vi "PROIECT4.vi"() -> ()   [LabVIEW 2021]
uses:
  <vilib>/express/express analysis/Spectral/Block/exnSpectralBlock spectral measurements RMS poly.vi
  <vilib>/express/express analysis/Spectral/Block/exnSpectralBlock spectral measurements RMS WFM.vi
  <vilib>/express/express analysis/Spectral/XNode/ExpressSpectralMeasurementsBlockNode.xnode
  <vilib>/measure/NI_MABase.lvlib
panel:
  in  "AMPLITUDINE":dbl(slide) scale=0.0..10.0
  in  "?":T1(radio)
  out "?":dbl
  out "?":dbl
  out "?":dbl
  out "GRAFIC SEMNAL":waveform(dbl)(graph)
  out "ANALIZA SPECTRALA":cluster{"f0":dbl, "df":dbl, "magnitude":dbl[]}(graph)
  in  "?":bool
  in  "FAZA":dbl(slide) scale=0.0..360.0
  in  "FRECVENTA":dbl(knob) scale=0.0..100.0
  # "amplitudine"
  # "faza"
  # "frecventa"
  # "ON/OFF"
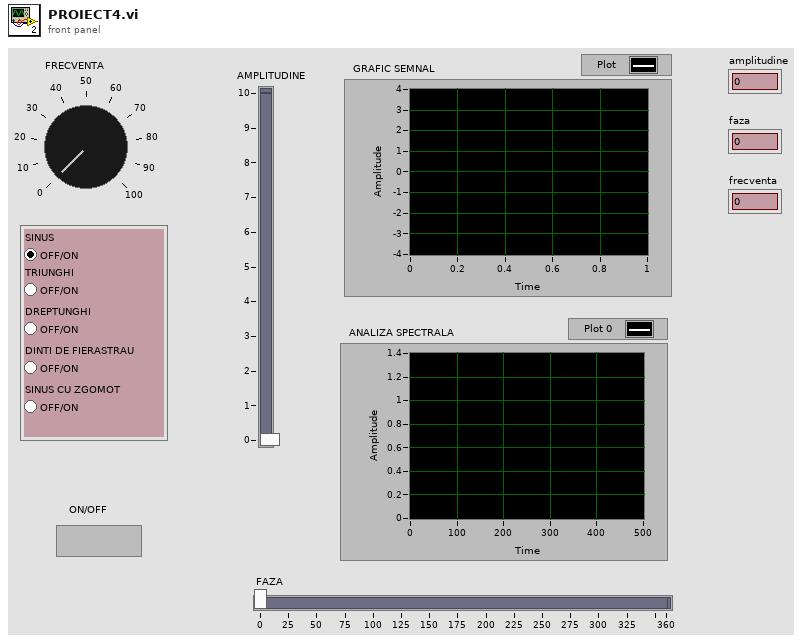
[diagram p1: front panel]
types:
  T1 = enum32{"SINUS", "TRIUNGHI", "DREPTUNGHI", "DINTI DE FIERASTRAU", "SINUS CU ZGOMOT"}
  T2 = cluster{"averaging mode":u16, "weighting mode":u16, "number of averages":u32}
  T3 = cluster{"dB On (F)":bool, "unwrap phase (F)":bool, "convert to degree (F)":bool}
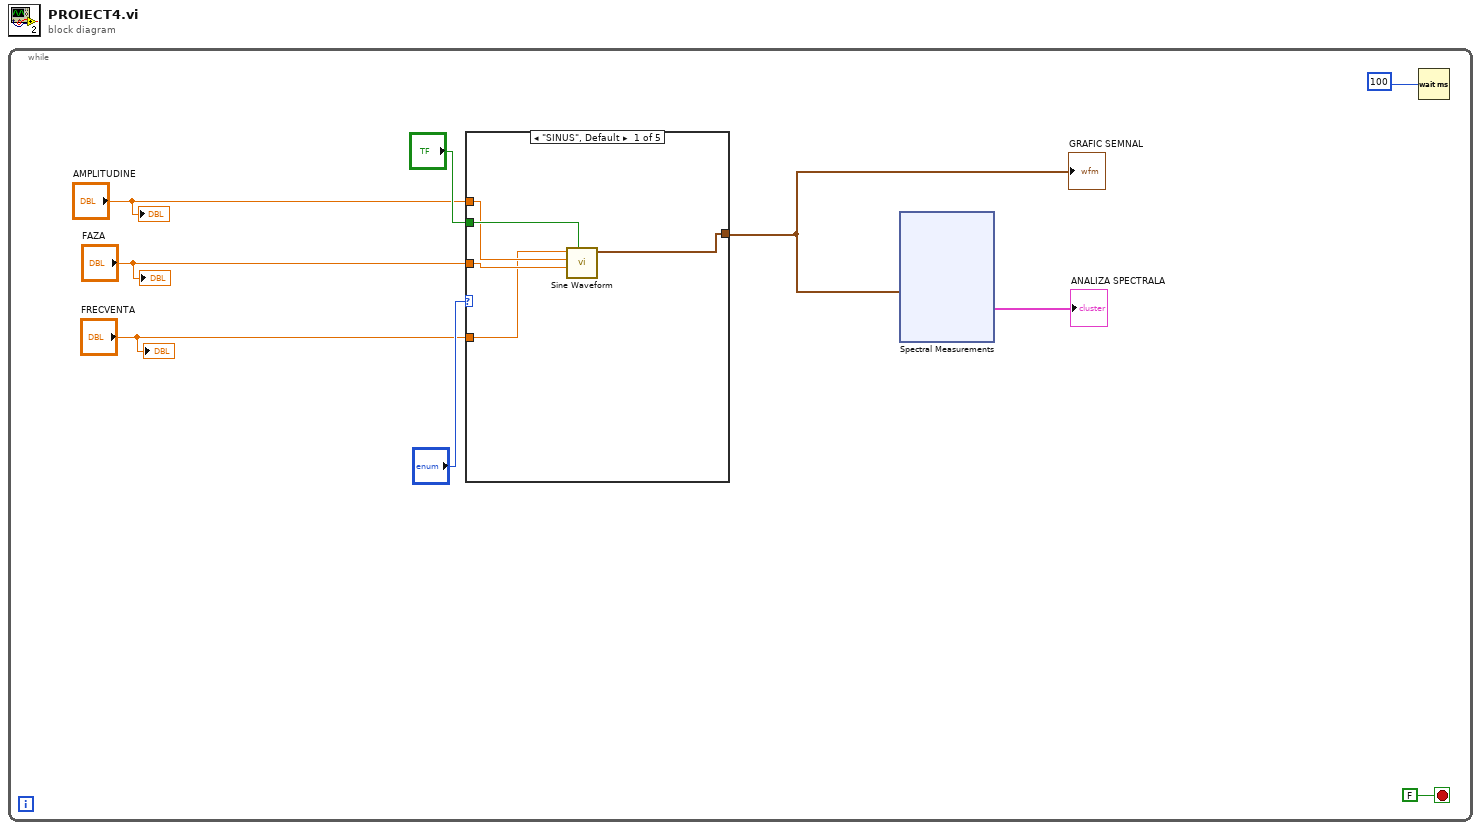
[diagram p0: block diagram]
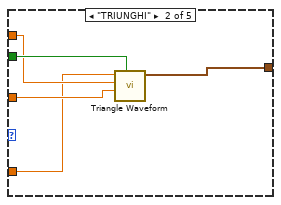
[diagram p2: hidden frame]
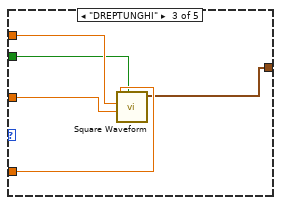
[diagram p3: hidden frame]
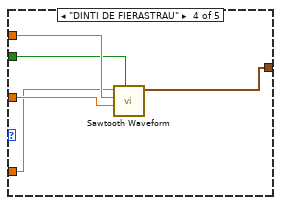
[diagram p4: hidden frame]
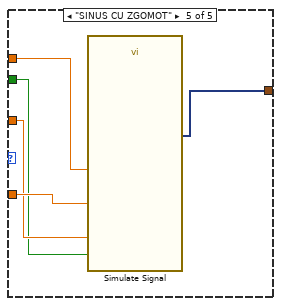
[diagram p5: hidden frame]
diagram:
  n1 = while {
    stop <- FALSE stop-if-true
    n2 = case shown="\"SINUS\", Default" "?" {
      tunnel: "FAZA" -> [w11 w16 w23 w28 w32]
      tunnel: "FRECVENTA" -> [w10 w15 w22 w27 w33]
      tunnel: "?" -> [w14 w18 w21 w26 w31]
      tunnel: [w13 w19 w20 w25 w30] -> w5
      tunnel: "AMPLITUDINE" -> [w12 w17 w24 w29 w34]
      frame "SINUS", Default {
        n3 = call <vilib>:"Sine Waveform.vi"("reset signal"=w14, "phase"=w11, "amplitude"=w12, "frequency"=w10) -> ("signal out"=w13:waveform(dbl))  [unwired: 6 in, 1 out]
      }
      frame "TRIUNGHI" {
        n4 = call <vilib>:"Triangle Waveform.vi"("reset signal"=w18, "phase"=w16, "amplitude"=w17, "frequency"=w15) -> ("signal out"=w19:waveform(dbl))  [unwired: 6 in, 1 out]
      }
      frame "DREPTUNGHI" {
        n5 = call <vilib>:"Square Waveform.vi"("reset signal"=w21, "phase"=w23, "amplitude"=w24, "frequency"=w22) -> ("signal out"=w20:waveform(dbl))  [unwired: 6 in, 1 out]
      }
      frame "DINTI DE FIERASTRAU" {
        n6 = call <vilib>:"Sawtooth Waveform.vi"("reset signal"=w26, "phase"=w28, "amplitude"=w29, "frequency"=w27) -> ("signal out"=w25:waveform(dbl))  [unwired: 6 in, 1 out]
      }
      frame "SINUS CU ZGOMOT" {
        n7 = call "Simulate Signal"("Reset Signal"=w31, "Frequency"=w33, "Amplitude"=w34, "Phase"=w32) -> ("Sine with Uniform Noise"=w30:dynamicdata)  [unwired: 10 in, 1 out]
      }
    }
    "GRAFIC SEMNAL" <- w5
    n8 = xnode "Spectral Measurements"("Signals"=w5) -> ("FFT - (RMS)"=→"ANALIZA SPECTRALA":cluster{"f0":dbl, "df":dbl, "magnitude":dbl[]})  [unwired: 1 in, 2 out]
    n9 = Wait (ms)(milliseconds to wait=u32 100 ("millisecond timer value")) -> ()  [unwired: 1 out]
    "?" <- "AMPLITUDINE"
    "?" <- "FAZA"
    "?" <- "FRECVENTA"
  }
